vi "Get All VI Data.vi"(8 "error in (no error)":errorcluster, 11 "Path":path) -> (0 "error out":errorcluster, 3 "VI Data":T1[](array[typedef]))   [LabVIEW 2023, in "VI Properties Editor.lvlib"]
doc: "Gets all VI data from <B>All Files in Dir</B>."
uses:
  VI Properties Editor.lvlib
  CTLs/VI Data.ctl
  CTLs/VI Properties.ctl
  <vilib>/picture/picture.llb/imagedata.ctl
  CTLs/Control Properties.ctl
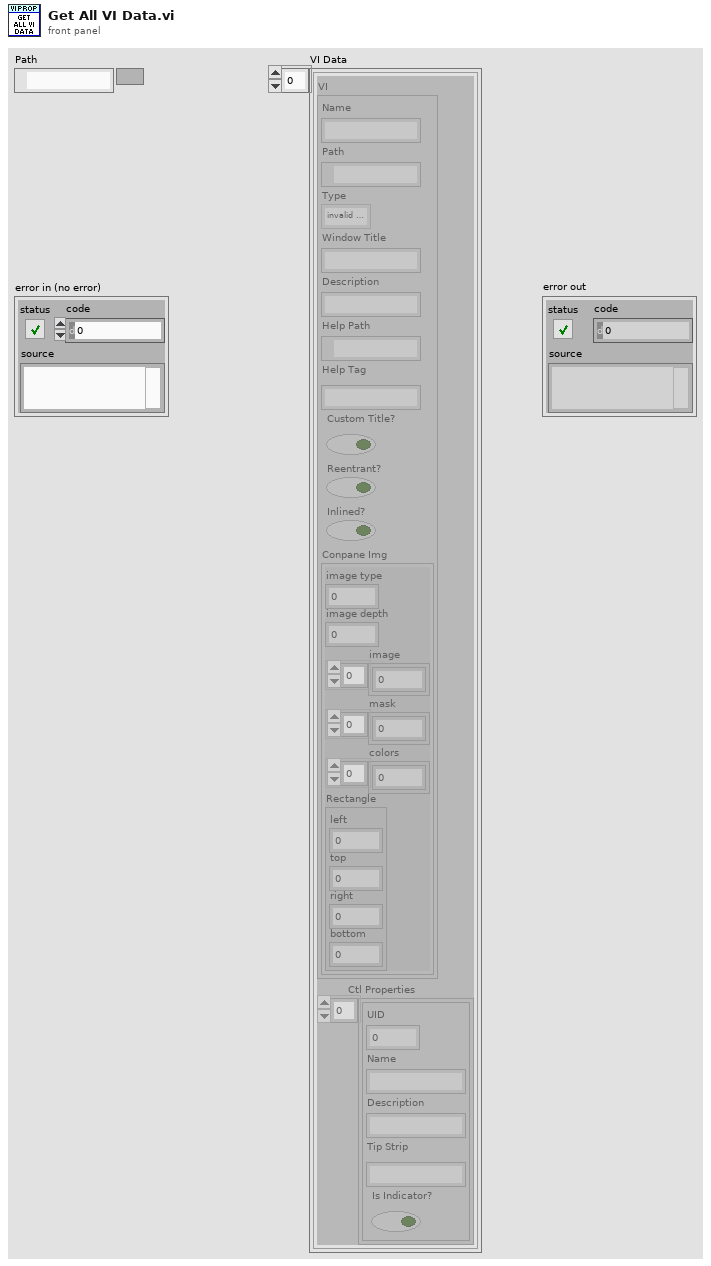
[diagram p1: front panel]
types:
  T1 = typedef "VI Properties Editor.lvlib/VI Data.ctl" = cluster{"VI":T2, "Ctl Properties":T4[]}
  T2 = typedef "VI Properties Editor.lvlib/VI Properties.ctl" = cluster{"Name":string, "Path":path, "Type":enum32{"invalid VI type", "Standard VI", "Control VI", "Global VI", "Polymorphic VI", "Configuration VI", "SubSystem", "Facade VI", "Method VI", "Statechart Diagram VI"}, "Window Title":string, "Description":string, "Help Path":path, "Help Tag":string, "Custom Title?":bool, "Reentrant?":bool, "Inlined?":bool, "Conpane Img":T3}
  T3 = typedef "imagedata.ctl" = cluster{"image type":i32, "image depth":i32, "image":u8[], "mask":u8[], "colors":u32[], "Rectangle":cluster{"left":i16, "top":i16, "right":i16, "bottom":i16}}
  T4 = typedef "VI Properties Editor.lvlib/Control Properties.ctl" = cluster{"UID":i32, "Name":string, "Description":string, "Tip Strip":string, "Is Indicator?":bool}
  T5 = enum32{"invalid VI type", "Standard VI", "Control VI", "Global VI", "Polymorphic VI", "Configuration VI", "SubSystem", "Facade VI", "Method VI", "Statechart Diagram VI"}
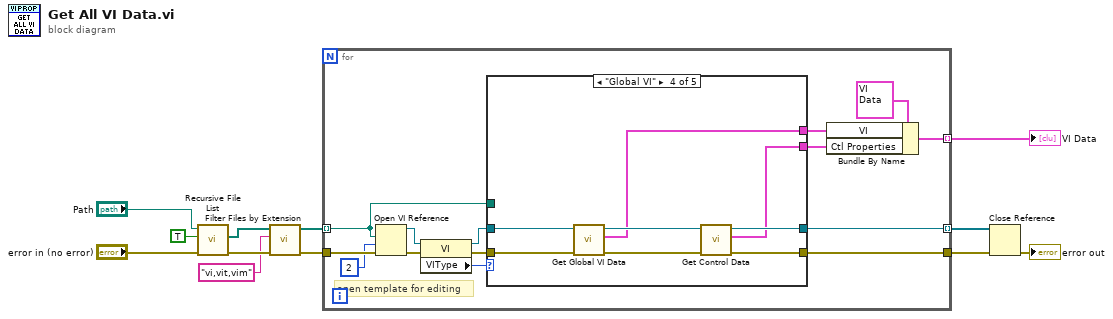
[diagram p0: block diagram]
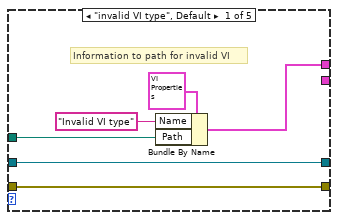
[diagram p2: hidden frame]
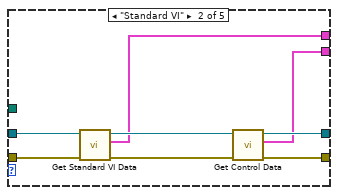
[diagram p3: hidden frame]
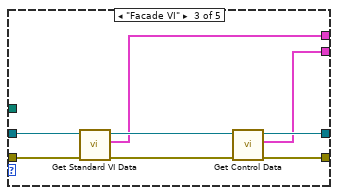
[diagram p4: hidden frame]
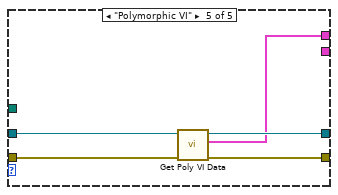
[diagram p5: hidden frame]
diagram:
  n1 = call <vilib>:"Recursive File List.vi"("error in (no error)"="error in (no error)", "Treat LLBs as Folders?"=TRUE, "Folder Path"="Path") -> ("error out"=w5:errorcluster, "All Files in Dir"=w3:path[])  [unwired: 4 in, 3 out]
  n2 = call "Filter Files by Extension.vi"("error in (no error)"=w5, "Extensions"="vi,vit,vim", "Files"=w3) -> ("error out"=w4:errorcluster, "Files out"=w2:path[])  [unwired: 7 in]
  n3 = for {
    tunnel: w2 -> [w18] mode=indexing
    tunnel: [w20] -> w10 mode=indexing
    tunnel: [w19] -> w12 mode=indexing
    tunnel: w4 -> [w25]
    tunnel: [w21] -> w11
    # "open template for editing"
    n4 = Open VI Reference(vi path=w18, options=2, error in (no error)=w25) -> (vi reference=w14:refnum<vi>, error out=w26:errorcluster)  [unwired: 3 in]
    n5 = property class="VI"(reference=w14, error in=w26) -> (reference out=w23:refnum<vi>, error out=w24:errorcluster, "VIType"=w22:T5)
    n6 = case shown="\"Global VI\"" w22 {
      tunnel: w24 -> [w32 w38 w46 w56 w57]
      tunnel: w23 -> [w31 w37 w45 w55 w58]
      tunnel: [w27 w34 w42 w49 w59] -> w15
      tunnel: [w32 w35 w43 w51 w61] -> w21
      tunnel: [w31 w39 w47 w52 w60] -> w20
      tunnel: w18 -> [w28 _ _ _ _]
      tunnel: [_ w33 w41 w50 _] -> w16
      frame "invalid VI type", Default {
        # "Information to path for invalid VI"
        n7 = Bundle By Name(cluster=T2 {"Name"="", "Path"=path "", "Type"=enum."invalid VI type", "Window Title"="", "Description"="", "Help Path"=path "", "Help Tag"="", "Custom Title?"=FALSE, "Reentrant?"=FALSE, "Inlined?"=FALSE, "Conpane Img"={"image type"=0, "image depth"=0, "image"=[], "mask"=[], "colors"=[], "Rectangle"={"left"=0, "top"=0, "right"=0, "bottom"=0}}} ("VI Properties"), "Name"="Invalid VI type" ("Help.Tag"), "Path"=w28) -> (w27:T2)
      }
      frame "Standard VI" {
        n8 = call "Get Standard VI Data.vi"("error in (no error)"=w38, "VI in"=w37) -> ("error out"=w36:errorcluster, "VI Properties"=w34:T2, "VI out"=w40:refnum<vi>)  [unwired: 7 in]
        n9 = call "Get Control Data.vi"("error in (no error)"=w36, "VI in"=w40) -> ("error out"=w35:errorcluster, "Control Data"=w33:T4[], "VI out"=w39:refnum<vi>)  [unwired: 7 in]
      }
      frame "Facade VI" {
        n10 = call "Get Standard VI Data.vi"("error in (no error)"=w46, "VI in"=w45) -> ("error out"=w44:errorcluster, "VI Properties"=w42:T2, "VI out"=w48:refnum<vi>)  [unwired: 7 in]
        n11 = call "Get Control Data.vi"("error in (no error)"=w44, "VI in"=w48) -> ("error out"=w43:errorcluster, "Control Data"=w41:T4[], "VI out"=w47:refnum<vi>)  [unwired: 7 in]
      }
      frame "Global VI" {
        n12 = call "Get Global VI Data.vi"("error in (no error)"=w56, "VI in"=w55) -> ("error out"=w54:errorcluster, "VI Properties"=w49:T2, "VI out"=w53:refnum<vi>)  [unwired: 7 in]
        n13 = call "Get Control Data.vi"("error in (no error)"=w54, "VI in"=w53) -> ("error out"=w51:errorcluster, "Control Data"=w50:T4[], "VI out"=w52:refnum<vi>)  [unwired: 7 in]
      }
      frame "Polymorphic VI" {
        n14 = call "Get Poly VI Data.vi"("error in (no error)"=w57, "VI in"=w58) -> ("error out"=w61:errorcluster, "VI Properties"=w59:T2, "VI out"=w60:refnum<vi>)  [unwired: 7 in]
      }
    }
    n15 = Bundle By Name(cluster=T1 {"VI"={"Name"="", "Path"=path "", "Type"=enum."invalid VI type", "Window Title"="", "Description"="", "Help Path"=path "", "Help Tag"="", "Custom Title?"=FALSE, "Reentrant?"=FALSE, "Inlined?"=FALSE, "Conpane Img"={"image type"=0, "image depth"=0, "image"=[], "mask"=[], "colors"=[], "Rectangle"={"left"=0, "top"=0, "right"=0, "bottom"=0}}}, "Ctl Properties"=[]}, "VI"=w15, "Ctl Properties"=w16) -> (w19:T1)
  }
  "VI Data" <- w12
  n16 = Close Reference(reference=w10, error in (no error)=w11) -> (error out=→"error out":errorcluster)
